vi "LoadVIsettings_flow.vi"(11 "VI path":path) -> ()   [LabVIEW 2011]
doc: "This VI uses Configuration File VIs to load the values of the controls of the VI you specify in VI path. LabVIEW uses the settings.dat file to load the values of the controls."
uses:
  <vilib>/Utility/config.llb/Read Key (String).vi
  <vilib>/Utility/config.llb/NI_LVConfig.lvlib
panel:
  # "Select Help»Show Context Help and move the cursor over the VI icon to display help for this VI."
  # "Instructions:\n1. Enter the path to settings.dat in the Configuration File path field.\n2. Enter the path to a VI with controls in the VI path field.\n3. Run the VI."
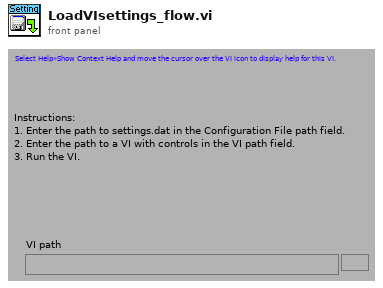
[diagram p1: front panel]
types:
  T1 = cluster{"name":string, "type desc":i16[], "flat data":string}[]
  T2 = typedef "NI_LVConfig.lvlib/Config Data RefNum.ctl" = refnum<k1>
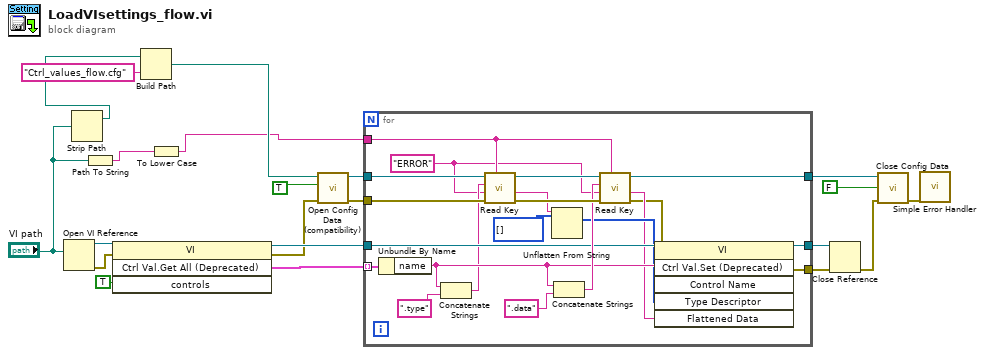
[diagram p0: block diagram]
diagram:
  n1 = Open VI Reference(vi path="VI path") -> (vi reference=w17:refnum<vi>, error out=w19:errorcluster)  [unwired: 5 in]
  n2 = Strip Path(path="VI path") -> (stripped path=w4:path)  [unwired: 1 out]
  n3 = Path To String(path="VI path") -> (string=w2:string)
  n4 = invoke class="VI" method="Ctrl Val.Get All (Deprecated)"(reference=w17, error in=w19, "controls"=TRUE) -> (reference out=w15:refnum<vi>, error out=w14:errorcluster, "Get All Control Values"=w20:T1)  [unwired: 1 in, 1 out]
  n5 = Build Path(base path=w4, name or relative path="Ctrl_values_flow.cfg") -> (appended path=w5:path)
  n6 = To Lower Case(string=w2) -> (all lower case string=w1:string)
  n7 = call <vilib>:"Open Config Data (compatibility).vi"("error in (no error)"=w14, "create file if necessary (T)"=TRUE ("create file if necessary? (T)"), "configuration file path"=w5) -> ("error out"=w13:errorcluster, "refnum"=w12:T2)  [unwired: 6 in, 1 out]
  n8 = for {
    tunnel: w20 -> [w42] mode=indexing
    tunnel: w1 -> [w35]
    tunnel: w15 -> [w33]
    tunnel: w13 -> [w40]
    tunnel: w12 -> [w41]
    tunnel: [w24] -> w11
    tunnel: [w23] -> w9
    tunnel: [w22] -> w8
    w30 = "ERROR" ("section")
    n9 = Unbundle By Name(w42) -> ("name"=w32:string)
    n10 = Concatenate Strings(w32, ".type" ("string")) -> (w31:string)
    n11 = call-poly <vilib>:"Read Key.vi"("section"=w35, "error in (no error)"=w40, "default value"=w30, "key"=w31, "refnum"=w41) -> ("error out"=w36:errorcluster, "value"=w29:string, "refnum out"=w37:T2)  [unwired: 3 in, 1 out]
    n12 = Unflatten From String(type=i16[] [] ("Array"), binary string=w29) -> (value=w27:i16[])  [unwired: 3 in, 2 out]
    n13 = Concatenate Strings(w32, ".data" ("string")) -> (w34:string)
    n14 = call-poly <vilib>:"Read Key.vi"("section"=w35, "error in (no error)"=w36, "default value"=w30, "key"=w34, "refnum"=w37) -> ("error out"=w25:errorcluster, "value"=w26:string, "refnum out"=w24:T2)  [unwired: 3 in, 1 out]
    n15 = invoke class="VI" method="Ctrl Val.Set (Deprecated)"(reference=w33, error in=w25, "Control Name"=w32, "Type Descriptor"=w27, "Flattened Data"=w26) -> (reference out=w23:refnum<vi>, error out=w22:errorcluster)  [unwired: 1 in, 4 out]
  }
  n16 = Close Reference(reference=w9, error in (no error)=w8) -> (error out=w7:errorcluster)
  n17 = call <vilib>:"Close Config Data.vi"("error in (no error)"=w7, "write file if changed (T)"=FALSE ("write configuration file? (T)"), "refnum"=w11) -> ("error out"=w21:errorcluster)  [unwired: 7 in, 1 out]
  n18 = call <vilib>:"Simple Error Handler.vi"("error in (no error)"=w21) -> ()  [unwired: 4 in, 5 out]
